vi "Add to Top Write.vi"(4 "error in (no error)":errorcluster, 5 "Value":bool, 6 "Container State":T3, 7 "Display State In":T1={"logTable"=refnum, "max items"=500, "displaydata"=[], "data"=[], "Auto Scroll"=TRUE, "current item"=500, "col headers"=[], "Add to Top"=TRUE, "Auto resize"=TRUE, "col size"=[], "filters"=[], "color cells"=[]}) -> (0 "error out":errorcluster, 3 "Display State Out":T1={"logTable"=refnum, "max items"=500, "displaydata"=[], "data"=[], "Auto Scroll"=TRUE, "current item"=500, "col headers"=[], "Add to Top"=TRUE, "Auto resize"=TRUE, "col size"=[], "filters"=[], "color cells"=[]})   [LabVIEW 2017, in "UI-DisplayTable(dev).xctl"]
uses:
  UI-DisplayTable(dev).xctl
  <vilib>/_xctls/Container State.ctl
  State.ctl
  Support/DEF-Filter.ctl
  <vilib>/_xctls/XControlSupport.lvlib
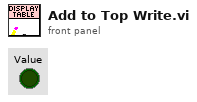
[diagram p1: front panel]
types:
  T1 = typedef "UI-DisplayTable(dev).xctl/State.ctl" = cluster{"logTable":refnum<vi>, "max items":i32, "displaydata":string[][], "data":string[][], "Auto Scroll":bool, "current item":i32, "col headers":string[], "Add to Top":bool, "Auto resize":bool, "col size":i32[], "filters":T2[], "color cells":cluster{"color cell":cluster{"Column":string, "Value":string, "Highlight Column":string}, "Color Box":u32}[]}
  T2 = typedef "UI-DisplayTable(dev).xctl/DEF-Filter.ctl" = cluster{"column":string, "value":string[]}
  T3 = typedef "XControlSupport.lvlib/Container State.ctl" = cluster{"Indicator?":bool, "Run Mode?":bool, " Refnum":refnum<vi>}
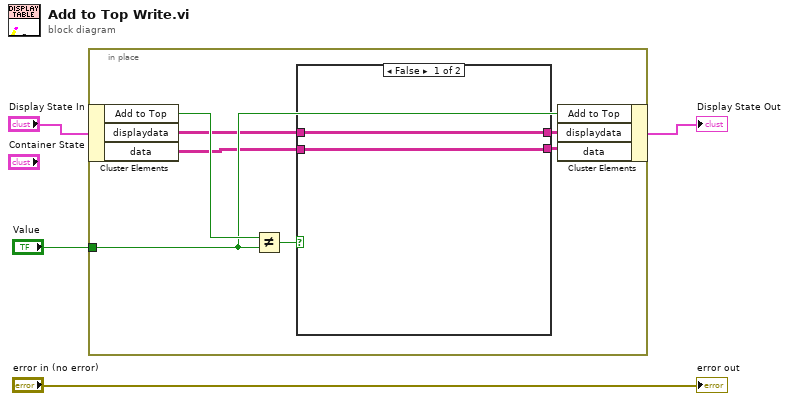
[diagram p0: block diagram]
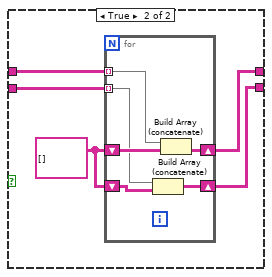
[diagram p2: hidden frame]
diagram:
  n1 = in-place {
    in-place-border: "Value" -> [w10]
    n2 = in-place-cluster #1("Display State In") -> ("Add to Top"=w11:bool, "displaydata"=w8:string[][], "data"=w6:string[][])
    n3 = Not Equal?(x=w11, y=w10) -> (x != y?=w9:bool)
    n4 = case shown="False" w9 {
      tunnel: w8 -> [w13 w17]
      tunnel: [w13 w18] -> w7
      tunnel: w6 -> [w12 w16]
      tunnel: [w12 w14] -> w5
      frame False {
      }
      frame True {
        w15 = string[][] [] ("displaydata")
        n5 = for {
          shift-right: [w23] -> w18
          shift-left: w15 -> [w24]
          tunnel: w17 -> [w22] mode=indexing
          tunnel: w16 -> [w19] mode=indexing
          shift-right: [w21] -> w14
          shift-left: w15 -> [w20]
          n6 = Build Array (concatenate)(w19, w20) -> (w21:string[][])
          n7 = Build Array (concatenate)(w22, w24) -> (w23:string[][])
        }
      }
    }
    n8 = in-place-cluster #1("Add to Top"=w10, "displaydata"=w7, "data"=w5) -> (→"Display State Out":T1)
  }
  "error out" <- "error in (no error)"
